vi "RGBclusterToColour.vi"(11 "RGBin":cluster{"R":dbl, "G":dbl, "B":dbl, "A":dbl}) -> (3 "colour":u32(colorbox))   [LabVIEW 2022 SP3]
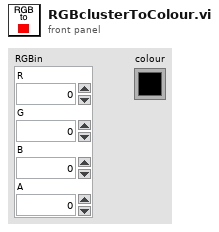
[diagram p1: front panel]
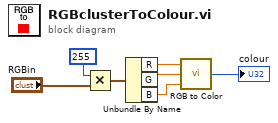
[diagram p0: block diagram]
diagram:
  n1 = Multiply(x=255, y="RGBin") -> (x*y=w2:cluster{"R":dbl, "G":dbl, "B":dbl, "A":dbl})
  n2 = Unbundle By Name(w2) -> ("R"=w4:dbl, "G"=w5:dbl, "B"=w6:dbl)
  n3 = call <vilib>:"RGB to Color.vi"("B"=w6, "G"=w5, "R"=w4) -> ("Color"=→"colour":u32)
